vi "Sierra - Frequency Drift test 3-9.vi"() -> ()   [LabVIEW 2015]
doc: "This VI demonstrates a simple procedure for setting up a spectrum analyzer, running an acquisition, and retrieving and plotting the waveform data.\n\nString indicators Binary WF Data and Sgl Float WF Data are initialized to empty strings. Waveform Graph is initialized to 0 for 100000 locations (just an arbitrary number for demonstration purposes).\n\ntkrsa6100 Initialize.vi opens the VISA Resource Name from the information entered by the user. It also presets the instrument by default to the Spectrum measurement. On completion it passes dup VISA Resource Name and error out to the following drivers.\n\nThe next VI to execute is tkrsa6100 Config Frequency.vi. Numeric control Center Freq (MHz)(50) is passed to the VI to set the center frequency to the default 50MHz value. The Set/Read Freq Setting (Set) is not wired since it defaults to SET, which is what is desired in this case. This is the case for all the configuration VI's in the example.\n\nThe next VI to execute is tkrsa6100 Config Spectrum Settings.vi. Enumerated control Spectrum Settings (CENTER FREQUENCY) is passed a Frequency Span constant and numeric control Freq Span (MHz) (40) to set the span to 40MHz.\n\nNext the reference level is set using tkrsa6100 Config RF Input.vi. Enumerated control Input Setting (REFERENCE LEVEL) is passed a Reference Level constant and numeric control Ref Level (dBm)(0) to set the reference level to 0dBm.\n\nNext the acquisition mode is set to single acquisition using tkrsa6100 Config Acquisition.vi. No parameters are passed since the default setting of this VI sets the acquisition mode to single.\n\nA single acquisition is then performed using tkrsa6100 Run Single Acquisition.vi. This VI sends an INIT command followed by a *OPC? Query. When the acquisition is completed the instrument returns a 1 and the next vi executes.\n\nThe binary waveform data is then retrieved by tkrsa6100 Spectrum Msmt Results.vi. The last acquisition data is retrieved by passing constant GET LAST ACQUISITION RESULT to enumerated input Run Acquisition and/or Get Result (RUN ACQUISITION & GET RESULT). The binary data is converted to a comma separated list of single precision floating point numbers by passing constant YES to enumerated input Convert Resp String (NO). The number of display points (total number of data bytes/4) is passed to a Spectral Display property node to scale the x axis of the graph. The binary data string from output Measurement Response String is copied to string indicator Binary WF Data. The converted binary data from output Converted Sgl Float Response String is copied to string indicator Sgl Float WF Data.\n\nSgl Float WF Data is then converted to an array by function Spreadsheet String to Array using a comma as the data separator. The output array is then passed to waveform graph Spectral Display for viewing.\n\nThe VISA Resource Name is closed using tkrsa6100 Close.vi."
panel:
  out "x/y 3":dbl
  in  "Combo Box":string(combo)
  out "Array 2":dbl[](array[numeric])
  out "x/y 2":dbl format="%#_15g"
  out "x-y":dbl
  in  "Trig Level (dBm)":dbl=-10.0 min=-170.0 max=50.0 step=0.1
  in  "VISA Resource Name":refnum<visa-resource-name>
  out "Sgl Float WF Data":string
  out "Binary WF Data":string
  out "Spectral Display":dbl[](graph)
  out "error out":errorcluster {"code" format="%#.0f"}
  # "Overview:  This VI  measures frequency drift by taking the average of the center frequencies of the first 25us of the packet (Preamble) and the last 25us of the packet (B-Field), \nand averaging their difference over 200 bursts.\nRequirements: RSA306 Spectrum Analyzer, Figure 31 test packet.\nInstructions: Select intrument identifier TCPIP0::127.0.0.1::inst0::INSTR under VISA Resource Name. Set trigger level to -10dBm (adjust as necessary depending on\nsignal strength). Select channel that the unit is operating at, under Combo Box."
  # "RSA6106A/6114A Acquire and Fetch\nSpectral Analysis Display"
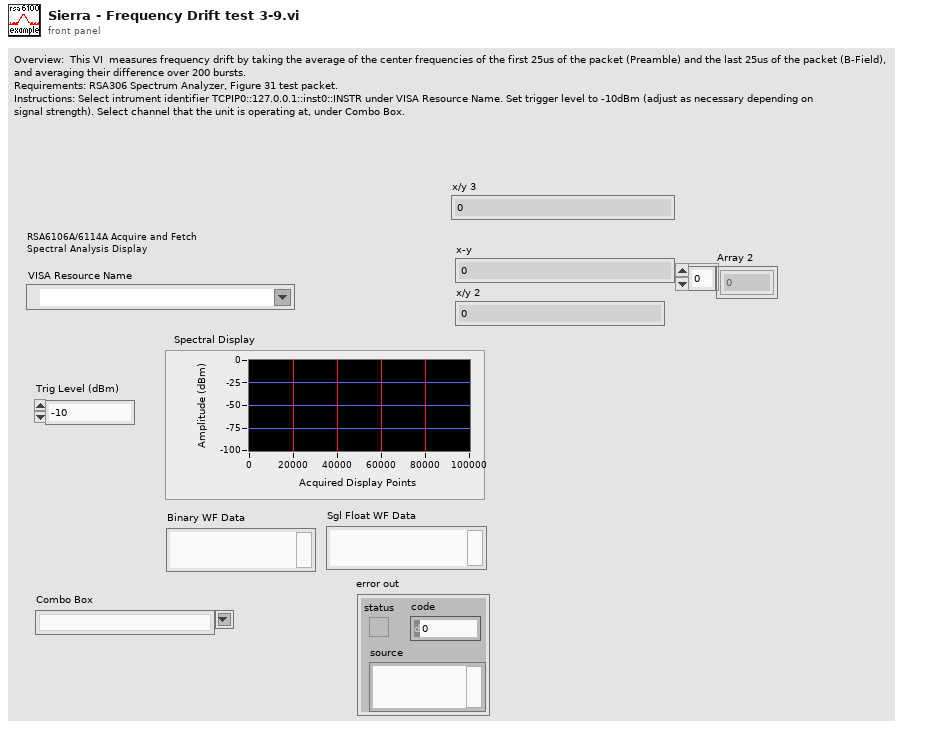
[diagram p1: front panel]
types:
  T1 = enum16{"CENTER FREQUENCY", "FREQUENCY SPAN", "RESOLUTION BW", "MAX REAL TIME SPAN (SET)", "START FREQUENCY", "STOP FREQUENCY", "FREQ STEP SIZE", "AUTO FREQ STEP ON", "AUTO FREQ STEP OFF", "AUTO RES BW ON", "AUTO RES BW OFF", "FFT WINDOW TYPE", "# POINTS", "RBW PROCESS ON", "RBW PROCESS OFF", "GAIN/BW OPTIMIZATION"}
  T2 = enum16{"RUN ACQUISITION  & GET RESULT", "GET LAST ACQUISITION RESULT"}
  T3 = enum16{"ANALYSIS REFERENCE", "ANALYSIS LENGTH", "ACTUAL ANALYSIS LENGTH (READ)", "AUTO ANALYSIS LENGTH ON", "AUTO ANALYSIS LENGTH OFF", "ANALYSIS OFFSET", "AUTO ANALYSIS OFFSET ON", "AUTO ANALYSIS OFFSET OFF", "SPECTRUM LENGTH", "ACTUAL SPECTRUM LENGTH (READ)", "AUTO SPECTRUM LENGTH ON", "AUTO SPECTRUM LENGTH OFF", "SPECTRUM OFFSET", "SPECTRUM TIME MODE", "DITHER MODE", "DITHER HW STATUS (READ)", "AUTO SPECTRUM OFFSETS AND ANALYSIS"}
  T4 = enum16{"TRIGGER SOURCE", "TRIGGER ON", "TRIGGER OFF", "TIME DELAY", "TIME POSITION", "TRIGGER EACH SEGMENT ON", "TRIGGER EACH SEGMENT OFF", "TRIGGER TYPE POWER", "TRIGGER TYPE FREQ MASK", "TRIGGER LEVEL", "TRIGGER SLOPE RISING", "TRIGGER SLOPE FALLING", "TDBW MODE ON", "TDBW MODE OFF", "TDBW", "ACTUAL TDBW (READ)", "CREATE NEW FMT (SET)", "SAVE FMT (SET)", "LOAD FMT (SET)", "FMT VIOLATION LOGIC", "FMT RBW AUTO", "FMT RBW MANUAL", "FMT RBW", "FORCE TRIGGER", "Trigger Position Auto"}
  T5 = enum16{"SPECTRUM ANALYZER", "DPSA", "SPECTROGRAM", "AMPL VS TIME", "FREQ VS TIME", "PHASE VS TIME", "IQ VS TIME", "TIME OVERVIEW"}
  T6 = enum16{"PEAK FIND (SET)", "NEXT PEAK LOWER (SET)", "NEXT PEAK HIGHER (SET)", "NEXT PEAK LEFT (SET)", "NEXT PEAK RIGHT (SET)", "MARKER TO CF (SET)", "MARKER TO TRACE", "MARKER FREQ", "MARKER AMPL (READ)", "DELTA MARKER FREQ (READ)", "DELTA MARKER AMPL (READ)"}
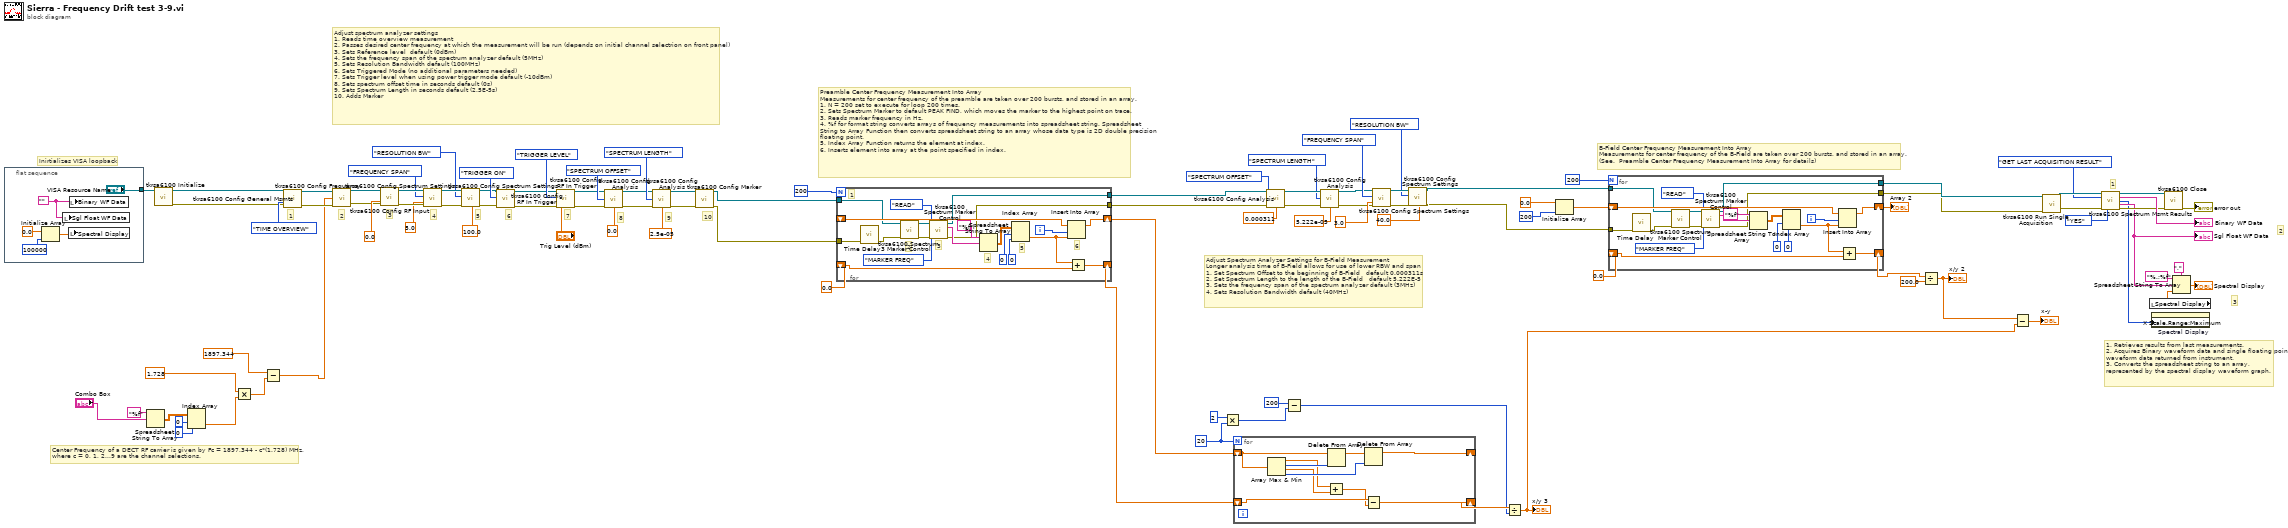
[diagram p0: block diagram]
diagram:
  w7 = 20
  # "3"
  # "2"
  # "1"
  # "1. Retrieves results from last measurements.\n2. Acquires Binary waveform data and single floating point waveform data returned from instrument.\n3. Converts the spreadsheet string to an array, represented by the spectral display waveform graph."
  # "B-Field Center Frequency Measurement Into Array\nMeasurements for center frequency of the B-Field are taken over 200 bursts, and stored in an array.\n(See.  Preamble Center Frequency Measurement Into Array for details)"
  # "Adjust Spectrum Analyzer Settings for B-Field Measurement\nLonger analysis time of B-Field allows for use of lower RBW and span\n1. Set Spectrum Offset to the beginning of B-Field   default 0.000311s\n2. Set Spectrum Length to the length of the B-Field   default 5.222E-5\n3. Sets the frequency span of the spectrum analyzer default (3MHz)\n4. Sets Resolution Bandwidth default (40MHz)"
  # "Preamble Center Frequency Measurement Into Array\nMeasurements for center frequency of the preamble are taken over 200 bursts, and stored in an array. \n1. N = 200 set to execute for loop 200 times.\n2. Sets Spectrum Marker to default PEAK FIND, which moves the marker to the highest point on trace.\n3. Reads marker frequency in Hz.\n4. %f for format string converts arrays of frequency measurements into spreadsheet string. Spreadsheet String to Array Function then converts spreadsheet string to an array whose data type is 2D double precision floating point. \n5. Index Array Function returns the element at index.\n6. Inserts element into array at the point specified in index."
  # "10"
  # "9"
  # "8"
  # "7"
  # "6"
  # "5"
  # "4"
  # "3"
  # "2"
  # "1"
  # "Adjust spectrum analyzer settings\n1. Reads time overview measurement \n2. Passes desired center frequency at which the measurement will be run (depends on initial channel selectrion on front panel)\n3. Sets Reference level  default (0dBm)\n4. Sets the frequency span of the spectrum analyzer default (5MHz)\n5. Sets Resolution Bandwidth default (100MHz)\n6. Sets Triggered Mode (no additional parameters needed)\n7. Sets Trigger level when using power trigger mode default (-10dBm)\n8. Sets spectrum offset time in seconds default (0s)\n9. Sets Spectrum Length in seconds default (2.5E-5s)\n10. Adds Marker"
  # "Inirtializes VISA loopback"
  # "Center Frequency of a DECT RF carrier is given by Fc = 1897.344 - c*(1.728) MHz, \nwhere c = 0, 1, 2...9 are the channel selections."
  n1 = flat-sequence {
    tunnel: ["VISA Resource Name"] -> w91
    frame #0 {
      w103 = ""
      n2 = Initialize Array(0.0 ("element"), 100000 ("dimension size")) -> (w105:dbl[])
      n3 = local write "Sgl Float WF Data"(w103) -> ()
      n4 = local write "Spectral Display"(w105) -> ()
      n5 = local write "Binary WF Data"(w103) -> ()
    }
  }
  n6 = Spreadsheet String To Array(format string="%f", spreadsheet string="Combo Box") -> (array=w15:dbl[][])  [unwired: 2 in]
  n7 = call <instrlib>:"tkrsa6100 Initialize.vi"("VISA Resource Name"=w91) -> ("dup VISA Resource Name"=w87:refnum<visa-resource-name>, "error out"=w88:errorcluster)  [unwired: 3 in, 10 out]
  n8 = Index Array(array=w15, index (row)=0, index (col)=0 ("disabled index (col)")) -> (element=w11:dbl)
  n9 = Multiply(x=1.728, y=w11) -> (x*y=w18:dbl)
  n10 = Subtract(x=1897.344, y=w18) -> (x-y=w17:dbl)
  n11 = call <instrlib>:"tkrsa6100 Config General Msmts.vi"("VISA Resource Name"=w87, "Measurement\n(SPECTRUM ANALYZER)"=T5."TIME OVERVIEW" ("Measurement\n(SPECTRUM ANALYZER)"), "error in (no error)"=w88) -> ("dup VISA Resource Name"=w72:refnum<visa-resource-name>, "error out"=w71:errorcluster)  [unwired: 10 in, 1 out]
  n12 = call <instrlib>:"tkrsa6100 Config Frequency.vi"("VISA Resource Name"=w72, "Msmt Freq (MHz)\n(1000)"=w17, "error in (no error)"=w71) -> ("dup VISA Resource Name"=w70:refnum<visa-resource-name>, "error out"=w69:errorcluster)  [unwired: 1 in, 10 out]
  n13 = call <instrlib>:"tkrsa6100 Config RF Input.vi"("VISA Resource Name"=w70, "Ref Level (0)"=0.0 ("Ref Level (dBm)(0)"), "error in (no error)"=w69) -> ("dup VISA Resource Name"=w62:refnum<visa-resource-name>, "error out"=w61:errorcluster)  [unwired: 4 in, 7 out]
  n14 = call <instrlib>:"tkrsa6100 Config Spectrum Settings.vi"("VISA Resource Name"=w62, "Spectrum Settings\n (CENTER FREQUENCY)"=T1."FREQUENCY SPAN" ("Spectrum Settings\n (CENTER FREQUENCY)"), "Freq Span\n(MHz)(40)"=5.0 ("Freq Span\n(MHz)(40)"), "error in (no error)"=w61) -> ("dup VISA Resource Name"=w55:refnum<visa-resource-name>, "error out"=w54:errorcluster)  [unwired: 13 in, 1 out]
  n15 = call <instrlib>:"tkrsa6100 Config Spectrum Settings.vi"("VISA Resource Name"=w55, "Spectrum Settings\n (CENTER FREQUENCY)"=T1."RESOLUTION BW" ("Spectrum Settings\n (CENTER FREQUENCY)"), "error in (no error)"=w54, "Res BW (KHz)\n(300)"=100.0 ("Res BW (KHz)\n(300)")) -> ("dup VISA Resource Name"=w53:refnum<visa-resource-name>, "error out"=w52:errorcluster)  [unwired: 13 in, 1 out]
  n16 = call <instrlib>:"tkrsa6100 Config RF In Trigger.vi"("VISA Resource Name"=w53, "Trigger Settings\n(TRIGGER SOURCE)"=T4."TRIGGER ON" ("Trigger Settings\n(TRIGGER SOURCE)"), "error in (no error)"=w52) -> ("dup VISA Resource Name"=w77:refnum<visa-resource-name>, "error out"=w78:errorcluster)  [unwired: 14 in, 1 out]
  n17 = call <instrlib>:"tkrsa6100 Config RF In Trigger.vi"("VISA Resource Name"=w77, "Trigger Settings\n(TRIGGER SOURCE)"=T4."TRIGGER LEVEL" ("Trigger Settings\n(TRIGGER SOURCE)"), "error in (no error)"=w78, "Trig Level\n(dBm)(-10)"="Trig Level (dBm)") -> ("dup VISA Resource Name"=w58:refnum<visa-resource-name>, "error out"=w57:errorcluster)  [unwired: 13 in, 1 out]
  n18 = call <instrlib>:"tkrsa6100 Config Analysis.vi"("VISA Resource Name"=w58, "Analysis Setting\n(ANALYSIS REFERENCE)"=T3."SPECTRUM OFFSET" ("Analysis Setting\n(ANALYSIS REFERENCE)"), "error in (no error)"=w57, "Offset Tme (S)(0)"=0.0) -> ("dup VISA Resource Name"=w75:refnum<visa-resource-name>, "error out"=w76:errorcluster)  [unwired: 9 in, 1 out]
  n19 = call <instrlib>:"tkrsa6100 Config Analysis.vi"("VISA Resource Name"=w75, "Length (S)(0.022)"=2.5e-05, "Analysis Setting\n(ANALYSIS REFERENCE)"=T3."SPECTRUM LENGTH" ("Analysis Setting\n(ANALYSIS REFERENCE)"), "error in (no error)"=w76) -> ("dup VISA Resource Name"=w49:refnum<visa-resource-name>, "error out"=w48:errorcluster)  [unwired: 9 in, 1 out]
  n20 = call <instrlib>:"tkrsa6100 Config Marker.vi"("VISA Resource Name"=w49, "error in (no error)"=w48) -> ("dup VISA Resource Name"=w38:refnum<visa-resource-name>, "error out"=w37:errorcluster)  [unwired: 11 in, 1 out]
  n21 = for {
    N: 200 ("Numeric") -> [_]
    shift-right: [w118] -> w9
    shift-left: _ -> [w117]
    tunnel: [w110] -> w35
    tunnel: [w113] -> w36
    tunnel: w38 -> [w112]
    tunnel: w37 -> [w111]
    shift-right: [w108] -> w8
    shift-left: 0.0 -> [w107]
    i -> [w116]
    # "1"
    # "6"
    # "5"
    # "4"
    # "3"
    # "2"
    n22 = call "Time Delay3"("error in (no error)"=w111) -> ("error out"=w120:errorcluster)  [unwired: 10 in]
    n23 = call <instrlib>:"tkrsa6100 Spectrum Marker Control.vi"("VISA Resource Name"=w112, "error in (no error)"=w120) -> ("dup VISA Resource Name"=w126:refnum<visa-resource-name>, "error out"=w119:errorcluster)  [unwired: 11 in, 1 out]
    n24 = call <instrlib>:"tkrsa6100 Spectrum Marker Control.vi"("VISA Resource Name"=w126, "Set/Read\nMarker Functions (SET)"=enum16{"SET", "READ"}."READ" ("Set/Read\nMarker Functions (SET)"), "Marker Function\n(PEAK FIND)"=T6."MARKER FREQ" ("Marker Function\n(PEAK FIND)"), "error in (no error)"=w119) -> ("dup VISA Resource Name"=w110:refnum<visa-resource-name>, "Marker\nResponse String"=w125:string, "error out"=w113:errorcluster)  [unwired: 9 in]
    n25 = Spreadsheet String To Array(format string="%f", spreadsheet string=w125) -> (array=w123:dbl[][])  [unwired: 2 in]
    n26 = Index Array(array=w123, index (row)=0, index (col)=0 ("disabled index (col)")) -> (element=w109:dbl)
    n27 = Insert Into Array(array=w117, index=w116, new element=w109) -> (w118:dbl[])
    n28 = Add(x=w109, y=w107) -> (x+y=w108:dbl)
  }
  n29 = Multiply(x=2, y=w7) -> (x*y=w3:i32)
  n30 = for {
    N: w7 -> [_]
    shift-right: [w132] -> _
    shift-left: w9 -> [w134]
    shift-right: [w127] -> w5
    shift-left: w8 -> [w129]
    n31 = Array Max & Min(array=w134) -> (max value=w131:dbl, max index (indices)=w136:i32, min value=w130:dbl, min index (indices)=w135:i32)
    n32 = Add(x=w131, y=w130) -> (x+y=w128:dbl)
    n33 = Delete From Array(array=w134, index=w136) -> (array with subset deleted=w133:dbl[])  [unwired: 1 in, 1 out]
    n34 = Delete From Array(array=w133, index=w135) -> (array with subset deleted=w132:dbl[])  [unwired: 1 in, 1 out]
    n35 = Subtract(x=w129, y=w128) -> (x-y=w127:dbl)
  }
  n36 = call <instrlib>:"tkrsa6100 Config Analysis.vi"("VISA Resource Name"=w35, "Analysis Setting\n(ANALYSIS REFERENCE)"=T3."SPECTRUM OFFSET" ("Analysis Setting\n(ANALYSIS REFERENCE)"), "error in (no error)"=w36, "Offset Tme (S)(0)"=0.000311) -> ("dup VISA Resource Name"=w66:refnum<visa-resource-name>, "error out"=w65:errorcluster)  [unwired: 9 in, 1 out]
  n37 = Subtract(x=200, y=w3) -> (x-y=w1:i32)
  n38 = call <instrlib>:"tkrsa6100 Config Analysis.vi"("VISA Resource Name"=w66, "Length (S)(0.022)"=5.222e-05, "Analysis Setting\n(ANALYSIS REFERENCE)"=T3."SPECTRUM LENGTH" ("Analysis Setting\n(ANALYSIS REFERENCE)"), "error in (no error)"=w65) -> ("dup VISA Resource Name"=w41:refnum<visa-resource-name>, "error out"=w40:errorcluster)  [unwired: 9 in, 1 out]
  n39 = call <instrlib>:"tkrsa6100 Config Spectrum Settings.vi"("VISA Resource Name"=w41, "Spectrum Settings\n (CENTER FREQUENCY)"=T1."FREQUENCY SPAN" ("Spectrum Settings\n (CENTER FREQUENCY)"), "Freq Span\n(MHz)(40)"=3.0 ("Freq Span\n(MHz)(40)"), "error in (no error)"=w40) -> ("dup VISA Resource Name"=w45:refnum<visa-resource-name>, "error out"=w44:errorcluster)  [unwired: 13 in, 1 out]
  n40 = call <instrlib>:"tkrsa6100 Config Spectrum Settings.vi"("VISA Resource Name"=w45, "Spectrum Settings\n (CENTER FREQUENCY)"=T1."RESOLUTION BW" ("Spectrum Settings\n (CENTER FREQUENCY)"), "error in (no error)"=w44, "Res BW (KHz)\n(300)"=40.0 ("Res BW (KHz)\n(300)")) -> ("dup VISA Resource Name"=w30:refnum<visa-resource-name>, "error out"=w29:errorcluster)  [unwired: 13 in, 1 out]
  n41 = Divide(x=w5, y=w1) -> (x/y=w4:dbl)
  "x/y 3" <- w4
  n42 = Initialize Array(0.0 ("element"), 200 ("dimension size")) -> (w31:dbl[])
  n43 = for {
    N: 200 ("Numeric") -> [_]
    shift-right: [w148] -> w22
    shift-left: w31 -> [w147]
    tunnel: [w140] -> w27
    tunnel: [w143] -> w26
    tunnel: w30 -> [w142]
    tunnel: w29 -> [w141]
    shift-right: [w138] -> w24
    shift-left: 0.0 -> [w137]
    i -> [w146]
    n44 = call "Time Delay"("error in (no error)"=w141) -> ("error out"=w150:errorcluster)  [unwired: 10 in]
    n45 = call <instrlib>:"tkrsa6100 Spectrum Marker Control.vi"("VISA Resource Name"=w142, "error in (no error)"=w150) -> ("dup VISA Resource Name"=w156:refnum<visa-resource-name>, "error out"=w149:errorcluster)  [unwired: 11 in, 1 out]
    n46 = call <instrlib>:"tkrsa6100 Spectrum Marker Control.vi"("VISA Resource Name"=w156, "Set/Read\nMarker Functions (SET)"=enum16{"SET", "READ"}."READ" ("Set/Read\nMarker Functions (SET)"), "Marker Function\n(PEAK FIND)"=T6."MARKER FREQ" ("Marker Function\n(PEAK FIND)"), "error in (no error)"=w149) -> ("dup VISA Resource Name"=w140:refnum<visa-resource-name>, "Marker\nResponse String"=w155:string, "error out"=w143:errorcluster)  [unwired: 9 in]
    n47 = Spreadsheet String To Array(format string="%f", spreadsheet string=w155) -> (array=w153:dbl[][])  [unwired: 2 in]
    n48 = Index Array(array=w153, index (row)=0, index (col)=0 ("disabled index (col)")) -> (element=w139:dbl)
    n49 = Insert Into Array(array=w147, index=w146, new element=w139) -> (w148:dbl[])
    n50 = Add(x=w139, y=w137) -> (x+y=w138:dbl)
  }
  "Array 2" <- w22
  n51 = Divide(x=w24, y=200.0) -> (x/y=w23:dbl)
  "x/y 2" <- w23
  n52 = Subtract(x=w23, y=w4) -> (x-y=→"x-y":dbl)
  n53 = call <instrlib>:"tkrsa6100 Run Single Acquisition.vi"("VISA Resource Name"=w27, "error in (no error)"=w26) -> ("dup VISA Resource Name"=w80:refnum<visa-resource-name>, "error out"=w79:errorcluster)  [unwired: 12 out]
  n54 = call <instrlib>:"tkrsa6100 Spectrum Msmt Results.vi"("VISA Resource Name"=w80, "Run Acquisition and/or \nGet Result (RUN ACQUISITION & GET RESULT)"=T2."GET LAST ACQUISITION RESULT" ("Run Acquisition and/or \nGet Result (RUN ACQUISITION & GET RESULT)"), "error in (no error)"=w79, "Convert Resp\nString(NO)"=enum16{"NO", "YES"}."YES" ("Convert Resp\nString(NO)")) -> ("dup VISA Resource Name"=w94:refnum<visa-resource-name>, "Measurement\nResponse String"=→"Binary WF Data":string, "# Data Points"=w92:i32, "Converted Sgl Float\nResponse String"=w93:string, "error out"=w96:errorcluster)  [unwired: 7 in]
  "Sgl Float WF Data" <- w93
  n55 = local read "Spectral Display"() -> (w101:dbl[])
  n56 = property on="Spectral Display" class="WFGraph (strict)"("X Scale.Range:Maximum"=w92) -> ()  [unwired: 2 in, 2 out]
  n57 = call <instrlib>:"tkrsa6100 Close.vi"("VISA Resource Name"=w94, "error in (no error)"=w96) -> ("error out"=→"error out":errorcluster)  [unwired: 13 out]
  n58 = Spreadsheet String To Array(delimiter (Tab)=",", format string="%.;%f", spreadsheet string=w93, array type (2D Dbl)=w101) -> (array=→"Spectral Display":dbl[])
